vi "Coord in Bounds.vi"(0 "Coords":T2, 2 "tolerance":dbl, 7 "Plot Bounds":T1, 11 "error in":errorcluster) -> (6 "position":T3 items=["Inside", "On Boundary", "Outside"], 15 "error out":errorcluster)   [LabVIEW 2021, in "ScrollZoomGraphChart.lvclass"]
uses:
  ScrollZoomGraphChart.lvclass
  <vilib>/Analysis/geometry.llb/Point in Polygon Position.ctl
  <vilib>/Utility/miscctls.llb/LVPoint32TypeDef.ctl
  <vilib>/Utility/miscctls.llb/LVRectTypeDef.ctl
  <vilib>/Analysis/geometry.llb/Point in Polygon (Scalar).vi
  <vilib>/Analysis/NI_AAL_Geometry.lvlib
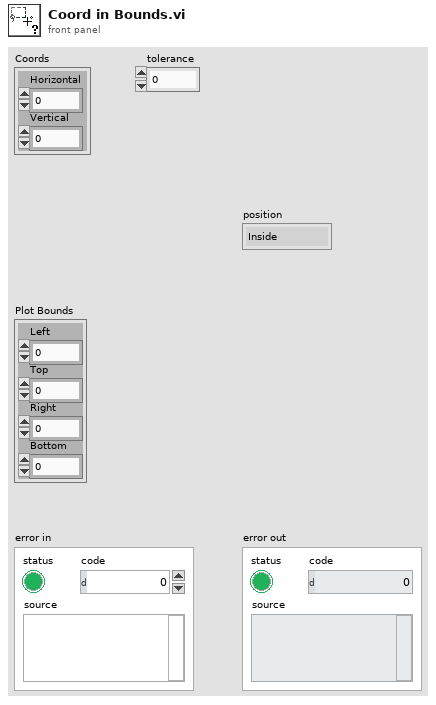
[diagram p1: front panel]
types:
  T1 = typedef "LVRectTypeDef.ctl" = cluster{"Left":i16, "Top":i16, "Right":i16, "Bottom":i16}
  T2 = typedef "LVPoint32TypeDef.ctl" = cluster{"Horizontal":i32, "Vertical":i32}
  T3 = typedef "NI_AAL_Geometry.lvlib/Point in Polygon Position.ctl" = u16
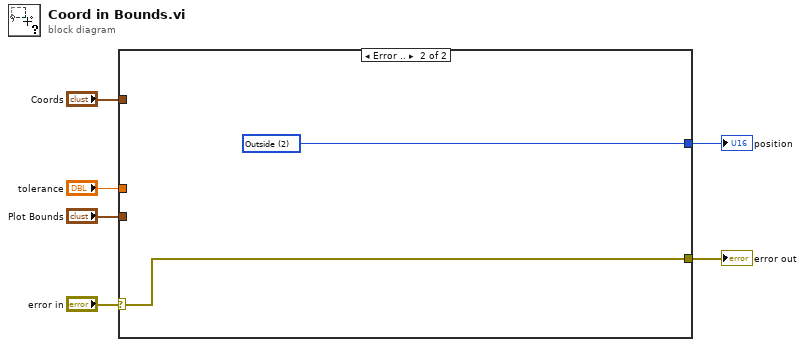
[diagram p0: block diagram]
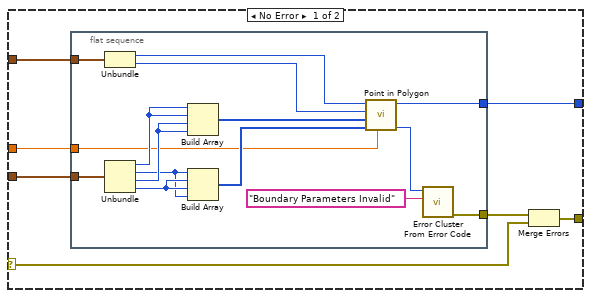
[diagram p2: hidden frame]
diagram:
  n1 = case shown="Error .." "error in" {
    selector: "error in" -> [w9 w29]
    tunnel: "tolerance" -> [w13 _]
    tunnel: [w12 w30] -> w5
    tunnel: "Coords" -> [w11 _]
    tunnel: "Plot Bounds" -> [w10 _]
    tunnel: [w8 w29] -> w1
    frame No Error {
      n2 = flat-sequence {
        tunnel: w10 -> [w28]
        tunnel: [w24] -> w12
        tunnel: w11 -> [w23]
        tunnel: w13 -> [w17]
        tunnel: [w15] -> w7
        frame #0 {
          n3 = Unbundle(w23) -> ("Horizontal"=w22:i32, "Vertical"=w21:i32)
          n4 = Unbundle(w28) -> ("Left"=w27:i16, "Top"=w18:i16, "Right"=w20:i16, "Bottom"=w19:i16)
          n5 = Build Array(w27, w27, w20, w20) -> (w26:i16[])
          n6 = Build Array(w18, w19, w19, w18) -> (w25:i16[])
          n7 = call-poly <vilib>:"Point in Polygon.vi"("tolerance"=w17, "Polygon Y"=w25, "Polygon X"=w26, "y"=w21, "x"=w22) -> ("error"=w16:i32, "position"=w24:T3)  [unwired: 5 in]
          n8 = call <vilib>:"Error Cluster From Error Code.vi"("error message (\"\")"="Boundary Parameters Invalid" ("error message (\"\")"), "error code (0)"=w16) -> ("error out"=w15:errorcluster)  [unwired: 7 in]
        }
      }
      n9 = Merge Errors(w7, w9) -> (w8:errorcluster)
    }
    frame Error {
      w30 = T3 2 items=["Inside", "On Boundary", "Outside"] ("position")
    }
  }
  "position" <- w5
  "error out" <- w1
